vi "Evaluate Stop Conditions.vi"(8 "Assert":bool, 9 "Index":i32, 10 "Complete":bool, 11 "Stop":bool) -> (0 "Asserted":bool, 1 "Index out":i32, 2 "Completed":bool, 3 "Stop out":bool)   [LabVIEW 2019, in "Test Executive.lvlib" / "Case Structure.lvclass"]
uses:
  <vilib>/gpm_packages/@cs/test-executive/Source/Test Executive/Case Structure/Case Structure.lvclass
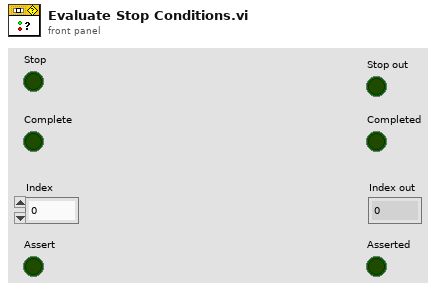
[diagram p1: front panel]
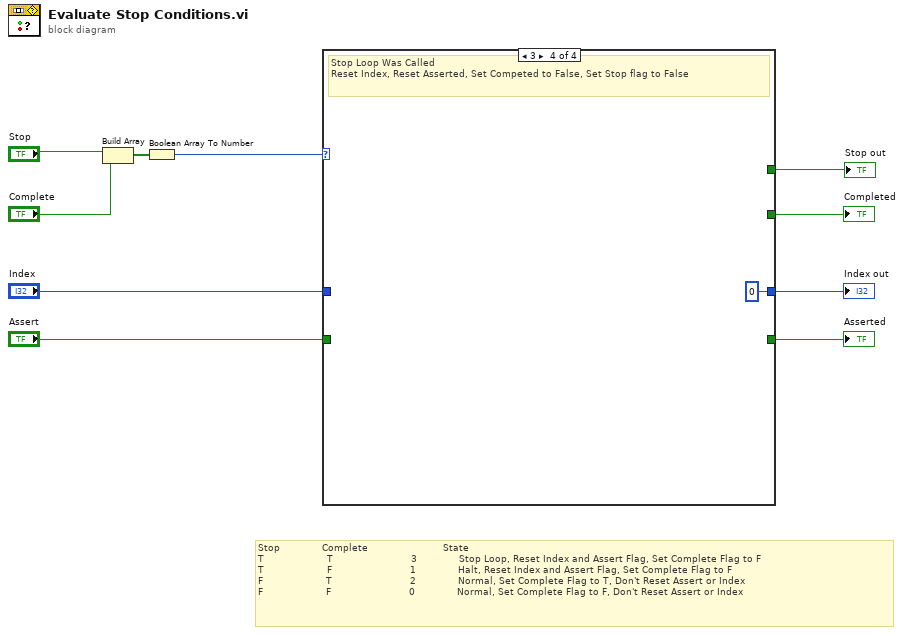
[diagram p0: block diagram]
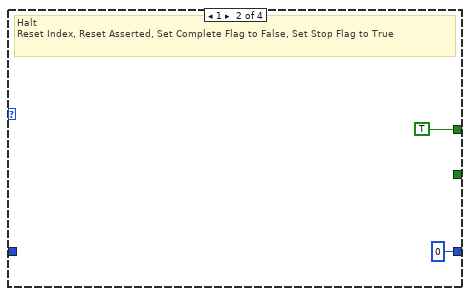
[diagram p3: hidden frame]
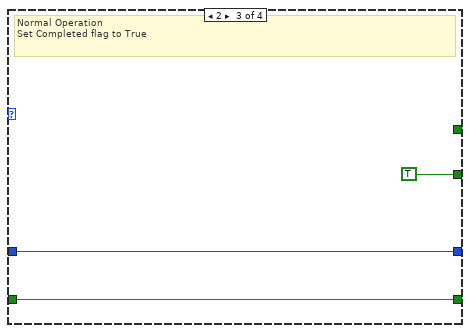
[diagram p4: hidden frame]
diagram:
  # "Stop              Complete                         State\nT                     T                          3              Stop Loop, Reset Index and Assert Flag, Set Complete Flag to F\nT                     F                          1              Halt, Reset Index and Assert Flag, Set Complete Flag to F\nF                     T                          2              Normal, Set Complete Flag to T, Don't Reset Assert or Index\nF                     F                          0              Normal, Set Complete Flag to F, Don't Reset Assert or Index"
  n1 = Build Array("Stop", "Complete") -> (w8:bool[])
  n2 = Boolean Array To Number(Boolean array=w8) -> (number=w7:u32)
  n3 = case shown="3" w7 {
    tunnel: "Index" -> [w12 _ w17 _]
    tunnel: "Assert" -> [w11 _ w16 _]
    tunnel: [w12 0 ("Index") w17 0 ("Index")] -> w4
    tunnel: [w11 _ w16 _] -> w3
    tunnel: [_ _ TRUE _] -> w2
    tunnel: [_ TRUE _ _] -> w1
    frame 0, Default {
      # "Normal Operation\nSet Completed flag to False"
    }
    frame 1 {
      # "Halt\nReset Index, Reset Asserted, Set Complete Flag to False, Set Stop Flag to True"
    }
    frame 2 {
      # "Normal Operation\nSet Completed flag to True"
    }
    frame 3 {
      # "Stop Loop Was Called\nReset Index, Reset Asserted, Set Competed to False, Set Stop flag to False"
    }
  }
  "Completed" <- w2
  "Index out" <- w4
  "Asserted" <- w3
  "Stop out" <- w1
